vi "ExternalInterfaceConfigurationToPlantUML.vi"() -> ()   [LabVIEW 2021]
uses:
  73289815-19b9-47e6-893a-c90994aa6943.vi
  <vilib>/JDP Science/JSONtext/JSON text to Variant.vi
  <vilib>/JDP Science/JSONtext/LVClass Serializer/JSONtext LVClass Serializer.lvclass
  <vilib>/JDP Science/JSONtext/Config Files/Config File.lvclass
panel:
  in  "TargetFolder":path=path "C:/Localdata/Projects/TriekselSoft/TriekselsoftApplicationFramework/Documentation"
  in  "ConfigFilePath":path=path "C:/Localdata/Projects/TriekselSoft/TriekselsoftApplicationFramework/ApplicationConfiguration/Mockup/InterfaceConfiguration.json"
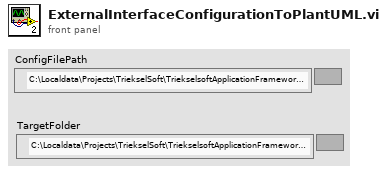
[diagram p1: front panel]
types:
  T1 = cluster{"Objects":cluster{"ObjectName":string, "ObjectType":string, "Interfaces":cluster{"Label":string, "ObjectName":string, "Type":string}[]}[]}
  T2 = cluster{"ObjectName":string, "ObjectType":string, "Interfaces":cluster{"Label":string, "ObjectName":string, "Type":string}[]}[]
  T3 = cluster{"Label":string, "ObjectName":string, "Type":string}[]
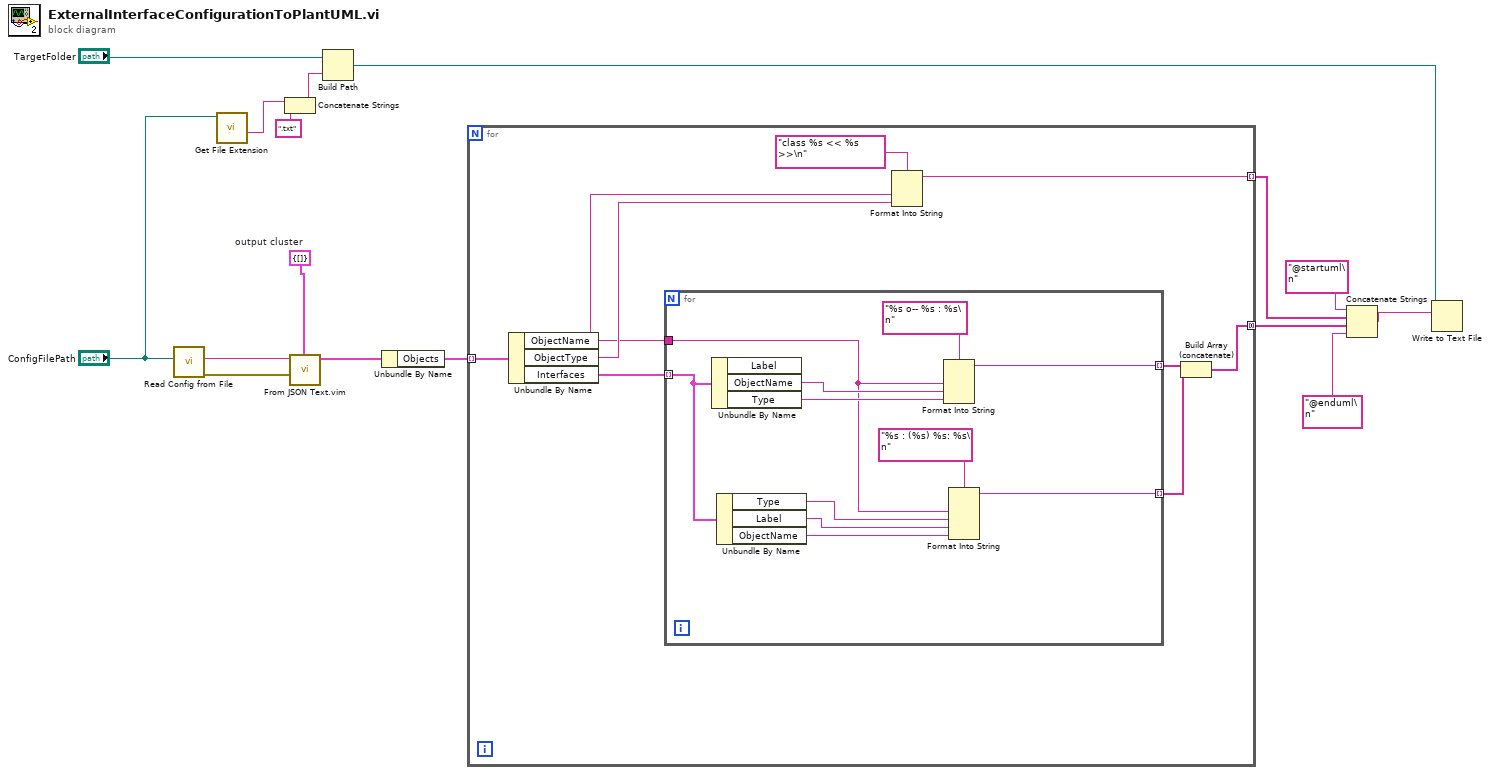
[diagram p0: block diagram]
diagram:
  w1 = T1 {"Objects"=[]}  # output cluster
  n1 = call <vilib>:"Read Config from File.vi"("config file path"="ConfigFilePath") -> ("error out"=w16:errorcluster, "<JSON>Config"=w15:string)  [unwired: 7 in, 2 out]
  n2 = call <vilib>:"Get File Extension.vi"("file"="ConfigFilePath") -> ("filename without extension"=w7:string)  [unwired: 6 in, 4 out]
  n3 = Concatenate Strings(w7, ".txt" ("string")) -> (w5:string)
  n4 = call "From JSON Text.vim"("Data Type and Default Value"=w1, "error in (no error)"=w16, "JSON"=w15) -> ("Data out"=w14:T1)  [unwired: 7 in, 1 out]
  n5 = Build Path(base path="TargetFolder", name or relative path=w5) -> (appended path=w4:path)
  n6 = Unbundle By Name(w14) -> ("Objects"=w13:T2)
  n7 = for {
    tunnel: w13 -> [w25] mode=indexing
    tunnel: [w21] -> w3 mode=indexing
    tunnel: [w18] -> w2 mode=concatenating
    n8 = Unbundle By Name(w25) -> ("ObjectName"=w20:string, "ObjectType"=w22:string, "Interfaces"=w24:T3)
    n9 = for {
      tunnel: w24 -> [w31] mode=indexing
      tunnel: w20 -> [w29]
      tunnel: [w34] -> w19 mode=indexing
      tunnel: [w30] -> w17 mode=indexing
      n10 = Unbundle By Name(w31) -> ("ObjectName"=w35:string, "Type"=w33:string)  [unwired: 1 out]
      n11 = Unbundle By Name(w31) -> ("Type"=w28:string, "Label"=w26:string, "ObjectName"=w27:string)
      n12 = Format Into String(format string="%s o-- %s : %s\n", w29, w35, w33) -> (resulting string=w34:string)  [unwired: 2 in, 1 out]
      n13 = Format Into String(format string="%s : (%s) %s: %s\n", w29, w28, w26, w27) -> (resulting string=w30:string)  [unwired: 2 in, 1 out]
    }
    n14 = Format Into String(format string="class %s << %s  >>\n", w20, w22) -> (resulting string=w21:string)  [unwired: 2 in, 1 out]
    n15 = Build Array (concatenate)(w19, w17) -> (w18:string[])
  }
  n16 = Concatenate Strings("@startuml\n" ("string"), w3, w2, "@enduml\n" ("string")) -> (w10:string)
  n17 = Write to Text File(file (use dialog)=w4, text=w10) -> ()  [unwired: 2 in, 3 out]
